vi "Database.Tools.ResultsParser(NaN).vi"(7 "Type":variant, 8 "error in (no error)":errorcluster, 9 "Results in":variant[][](array[variant])) -> (0 "error out":errorcluster, 3 "Results out":variant[][](array[variant]))   [LabVIEW 2016]
uses:
  <vilib>/Utility/VariantDataType/Type.ctl
  <vilib>/Utility/VariantDataType/VariantType.lvlib
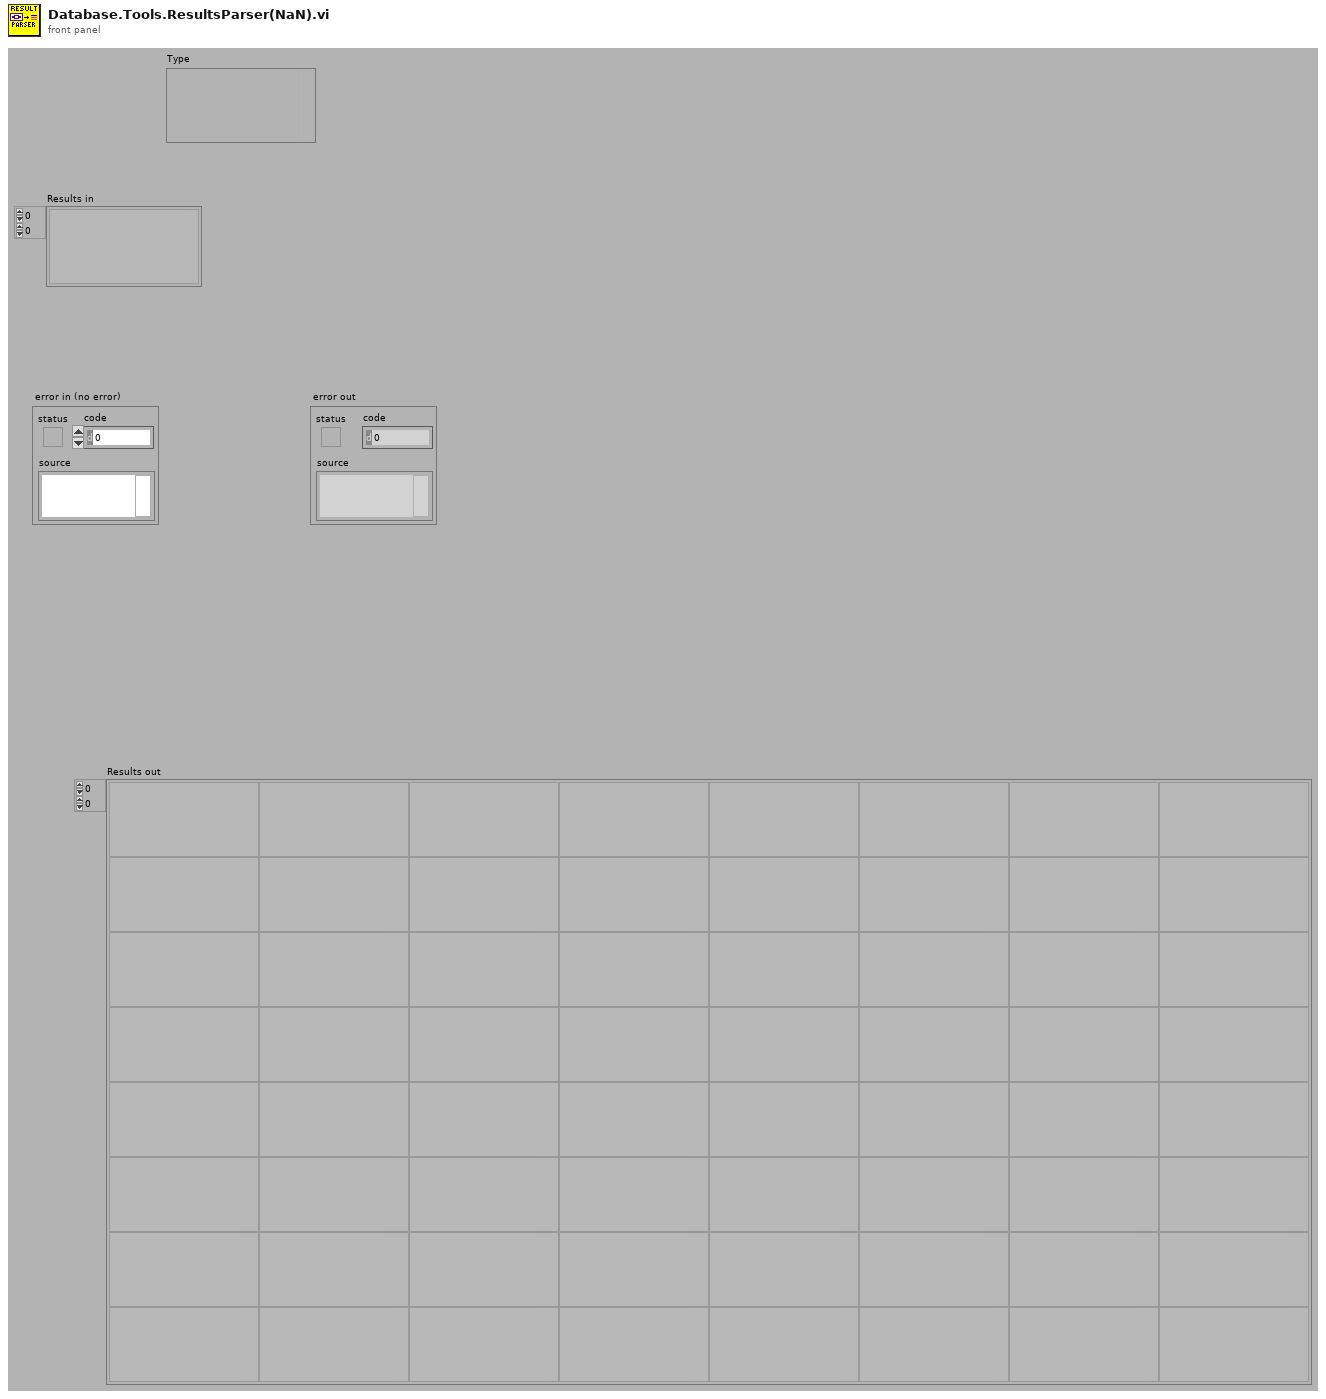
[diagram p1: front panel]
types:
  T1 = typedef "Database Connectivity Toolkit.lvlib/DB Tools LV Type.ctl" = enum16{"Unsupported", "Boolean", "I8", "I16", "I32", "U8", "U16", "U32", "SGL", "DBL", "EXT", "CSG", "CDB", "CXT", "String", "Path", "Picture", "I/O Channel", "Array", "Cluster", "Variant", "WDT"}
  T2 = typedef "VariantType.lvlib/Type.ctl" = enum8{"Invalid Type", "Void", "I8", "I16", "I32", "I64", "U8", "U16", "U32", "U64", "Single Float", "Double Float", "Extended Float", "Single Complex", "Double Complex", "Extended Complex", "Enum U8", "Enum U16", "Enum U32", "Enum U64", "Single Float With Unit", "Double Float With Unit", "Extended Float With Unit", "Single Complex with Unit", "Double Complex with Unit", "Extended Complex with Unit", "Boolean", "String", "Path", "Picture", "Tag", "Array", "Cluster", "Variant", "LV Variant", "Waveform", "Timestamp", "Digital Waveform", "Digital Data", "ExpressData", "Refnum", "External Data", "VI", "Poly VI", "LabVIEW Class Instance", "Fixed Point"}
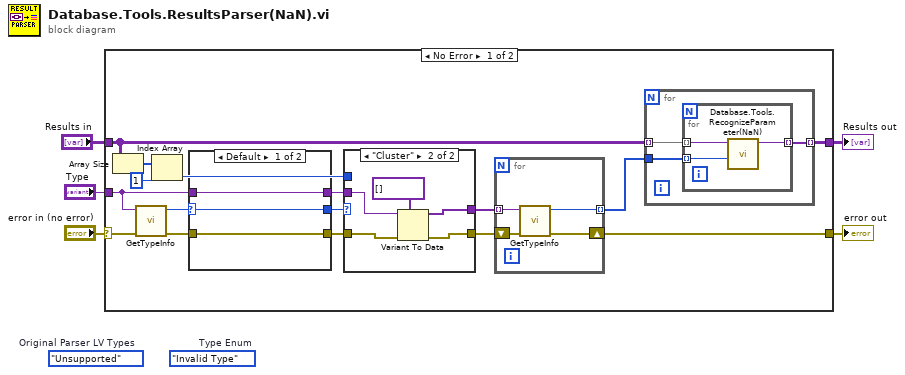
[diagram p0: block diagram]
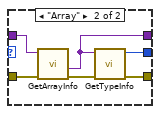
[diagram p2: hidden frame]
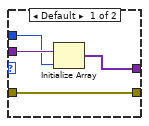
[diagram p3: hidden frame]
diagram:
  (unwired) DB_Tools_LV_Type."Unsupported"  # Original Parser LV Types
  (unwired) Type."Invalid Type"  # Type Enum
  n1 = case shown="No Error" "error in (no error)" {
    selector: "error in (no error)" -> [w20 w51]
    tunnel: [w17 w51] -> w4
    tunnel: "Type" -> [w21 _]
    tunnel: "Results in" -> [w16 w50]
    tunnel: [w18 w50] -> w1
    frame No Error {
      n2 = Array Size(array=w16) -> (size(s)=w8:i32[])
      n3 = call <vilib>:"GetTypeInfo.vi"("error in (no error)"=w20, "Variant"=w21) -> ("error out"=w15:errorcluster, "Type Enum"=w11:T2)  [unwired: 5 in, 3 out]
      n4 = Index Array(array=w8, index=1) -> (element=w6:i32)
      n5 = case shown="Default" w11 {
        selector: w11 -> [w27 _]
        tunnel: w21 -> [w28 w29]
        tunnel: w15 -> [w26 w34]
        tunnel: [w26 w32] -> w14
        tunnel: [w28 w31] -> w13
        tunnel: [w27 w30] -> w12
        frame Default {
        }
        frame "Array" {
          n6 = call <vilib>:"GetArrayInfo.vi"("error in (no error)"=w34, "Variant"=w29) -> ("error out"=w33:errorcluster, "ArrayElement"=w31:variant)  [unwired: 6 in, 2 out]
          n7 = call <vilib>:"GetTypeInfo.vi"("error in (no error)"=w33, "Variant"=w31) -> ("error out"=w32:errorcluster, "Type Enum"=w30:T2)  [unwired: 5 in, 3 out]
        }
      }
      n8 = case shown="\"Cluster\"" w12 {
        tunnel: w14 -> [w38 w43]
        tunnel: [w38 w42] -> w10
        tunnel: w13 -> [w37 w40]
        tunnel: [w35 w39] -> w9
        tunnel: w6 -> [w36 _]
        frame Default {
          n9 = Initialize Array(w37, w36) -> (w35:variant[])
        }
        frame "Cluster" {
          n10 = Variant To Data(error in=w43, type=variant[] [], Variant=w40) -> (data=w39:variant[], error out=w42:errorcluster)
        }
      }
      n11 = for {
        tunnel: w9 -> [w24] mode=indexing
        tunnel: [w23] -> w19 mode=indexing
        shift-right: [w22] -> w17
        shift-left: w10 -> [w25]
        n12 = call <vilib>:"GetTypeInfo.vi"("error in (no error)"=w25, "Variant"=w24) -> ("error out"=w22:errorcluster, "Type Enum"=w23:T2)  [unwired: 5 in, 3 out]
      }
      n13 = for {
        tunnel: w19 -> [w46]
        tunnel: w16 -> [w45] mode=indexing
        tunnel: [w44] -> w18 mode=indexing
        n14 = for {
          tunnel: w46 -> [w47] mode=indexing
          tunnel: w45 -> [w49] mode=indexing
          tunnel: [w48] -> w44 mode=indexing
          n15 = call "Database.Tools.RecognizeParameter(NaN).vi"("Type Enum"=w47, "Variant data in"=w49) -> ("Variant data out"=w48:variant)  [unwired: 9 in]
        }
      }
    }
    frame Error {
    }
  }
  "error out" <- w4
  "Results out" <- w1
